vi "Dequeue Action.vi"(8 "error in (no error)":errorcluster, 10 "Wait? (F)":bool) -> (0 "error out":errorcluster, 2 "element":T1)   [LabVIEW 2014]
uses:
  Action/Action.ctl
  Action/Action Priority.ctl
  Action/Action Name.ctl
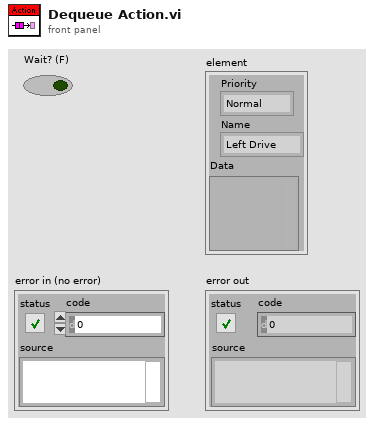
[diagram p1: front panel]
types:
  T1 = typedef "Action.ctl" = cluster{"Priority":T2, "Name":T3, "Data":variant}
  T2 = typedef "Action Priority.ctl" = enum16{"Normal", "High", "Interrupt"}
  T3 = typedef "Action Name.ctl" = enum16{"Left Drive", "Right Drive", "Half Drive", "Straight Drive"}
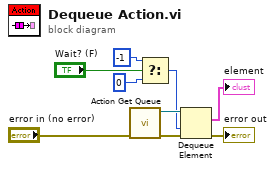
[diagram p0: block diagram]
diagram:
  n1 = call "Action Get Queue.vi"("error in (no error)"="error in (no error)") -> ("error out"=w6:errorcluster, "queue out"=w8:refnum<queue>)  [unwired: 9 in]
  n2 = Select(t=-1, s="Wait? (F)", f=0) -> (s? t:f=w3:i32)
  n3 = Dequeue Element(queue=w8, timeout in ms (-1)=w3, error in (no error)=w6) -> (element=→"element":T1, error out=→"error out":errorcluster)  [unwired: 2 out]
